vi "EAGLE Setup Screen V2.vi"() -> (1 "Table Control":string[][](table))   [LabVIEW 2015]
panel:
  in  "AvgPuls":dbl=0.3 min=0.3 max=2.0 format="%#.2g"
  in  "DfromLim":dbl min=-1000.0 max=1000.0
  in  "TbetweenP":u32=4 min=4 max=10
  in  "NumOfLas":u32=1 min=1 max=100
  in  "EyeColor":enum32{"Dark", "Blue/Green"}(radio) caption="Eye Color"
  in  "EyeSelect":enum32{"Right Eye", "Left Eye"}(radio) caption="Eye"
  in  "TreatArea":enum32{"Upper 180", "Lower 180", "Full 360"}(radio) caption="Treatment Area"
  in  "ID":string caption="Patient ID"
  in  "Save":bool
  in  "AvgPulseEn":dbl(slide)=1.0 caption="Average Pulse\nEnergy [mJ]" min=0.3 max=2.0 step=0.1 scale=0.3..2.0
  in  "DisFromLimbus":dbl(slide)=1.0 caption="Distance From \nLimbus [um]" min=-1000.0 max=1000.0 step=0.1 scale=-1000.0..1000.0
  in  "TBetweenPulses":u8(slide)=4 caption="Time Between \nPulses [mSec]" min=4 max=10 step=1 scale=4.0..10.0
  in  "LaserShots":u8(slide)=1 caption="Number of \nLaser Pulses" min=1 max=100 step=1 scale=1.0..100.0
  in  "FillSetupList":bool
  in  "Done":bool
  # "Treatment Settings"
  # "Laser Settings"
  # "Eye Info"
  # "Treatment Info"
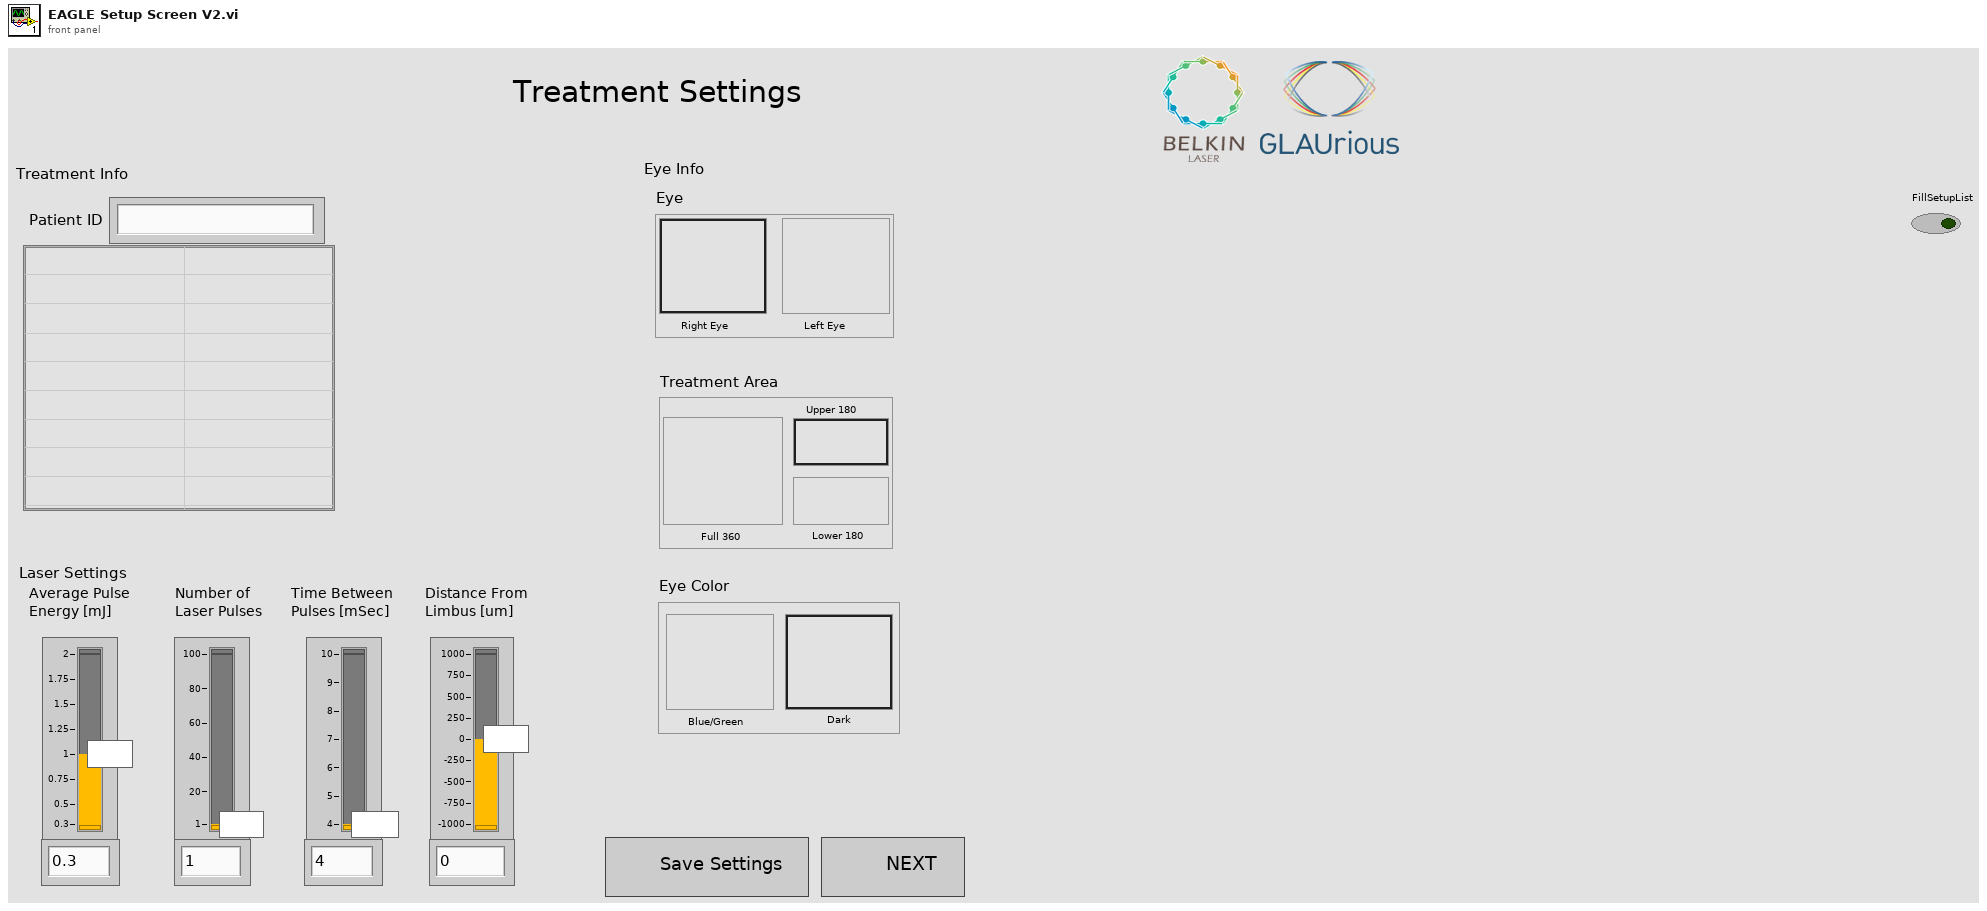
[diagram p1: front panel]
types:
  T1 = typedef "LVRectTypeDef.ctl" = cluster{"Left":i16, "Top":i16, "Right":i16, "Bottom":i16}
  T2 = typedef "LVPositionTypeDef.ctl" = cluster{"Left":i32, "Top":i32}
  T3 = cluster{"EyeSelect":enum32{"Right Eye", "Left Eye"}, "TBetweenPulses":u8, "LaserShots":u8, "TreatArea":enum32{"Upper 180", "Lower 180", "Full 360"}, "DisFromLimbus":dbl, "ID":string, "EyeColor":enum32{"Dark", "Blue/Green"}, "AvgPulseEn":dbl}
  T4 = cluster{"EyeSelect":enum32{"Right Eye", "Left Eye"}, "TBetweenPulses":u8, "LaserShots":u8, "TreatArea":enum32{"Upper 180", "Lower 180", "Full 360"}, "DisFromLimbus":dbl, "ID":string, "EyeColor":enum32{"Dark", "Blue/Green"}, "AvgPulse":dbl}
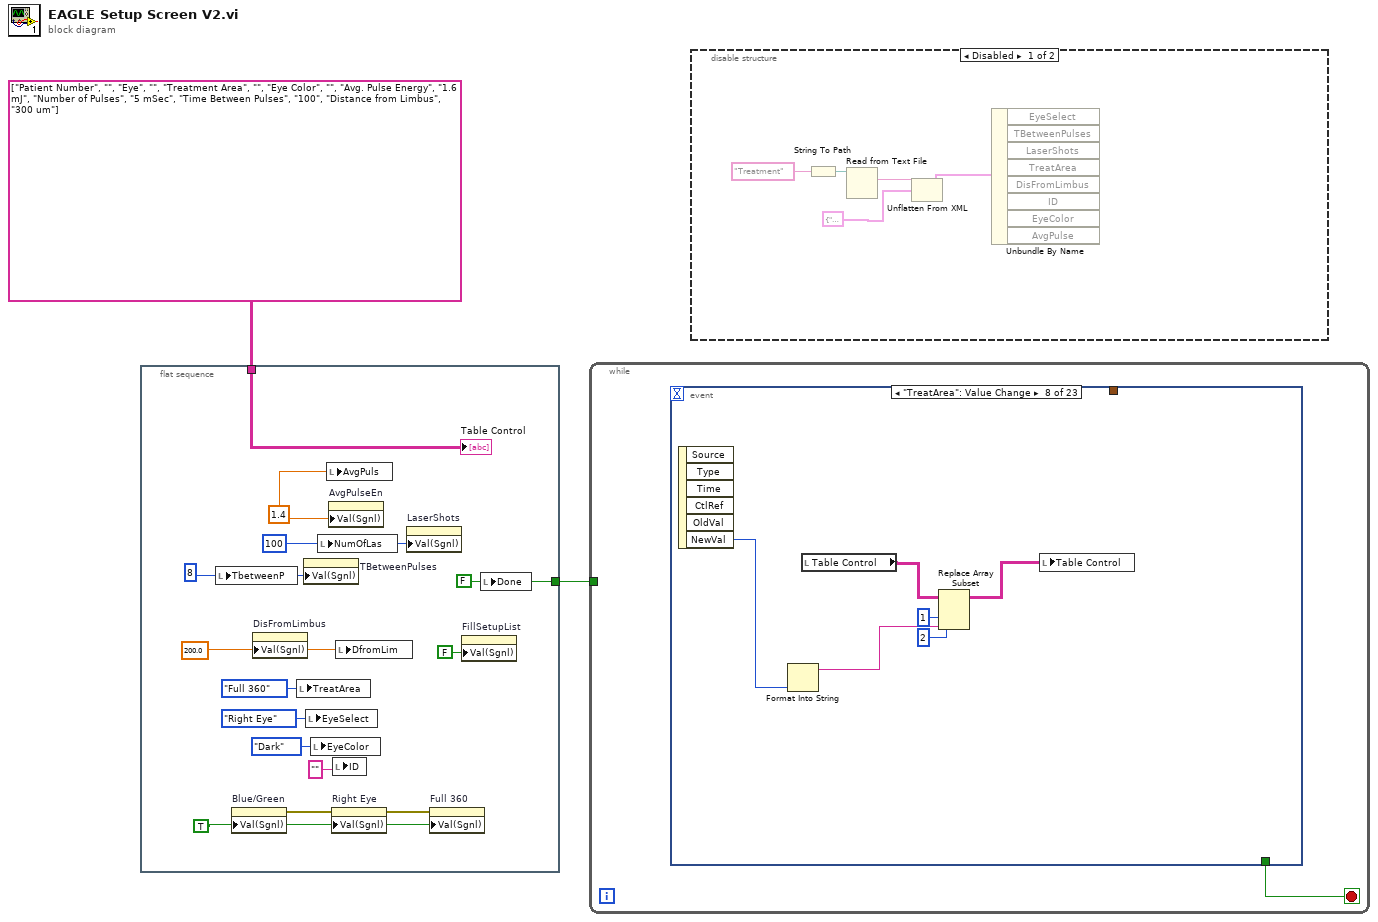
[diagram p0: block diagram]
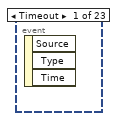
[diagram p3: hidden frame]
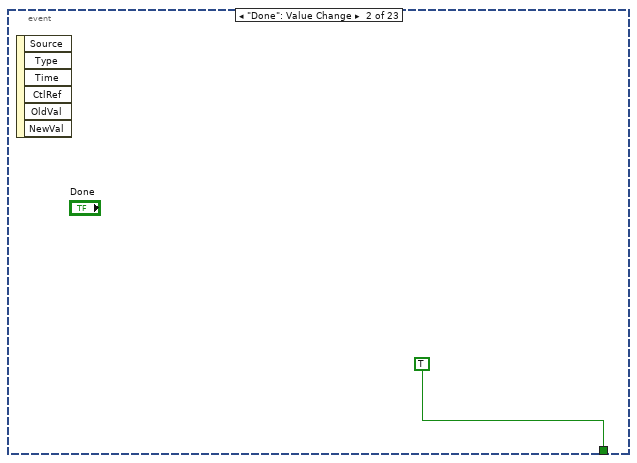
[diagram p4: hidden frame]
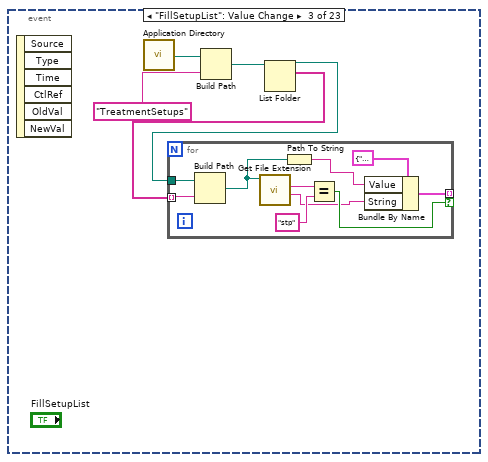
[diagram p5: hidden frame]
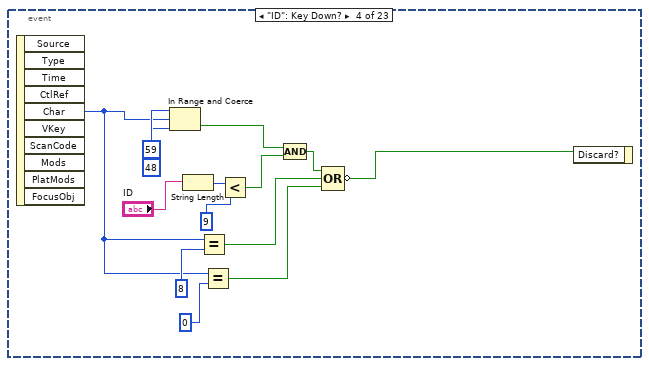
[diagram p6: hidden frame]
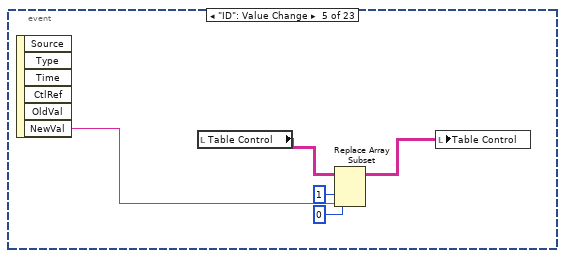
[diagram p7: hidden frame]
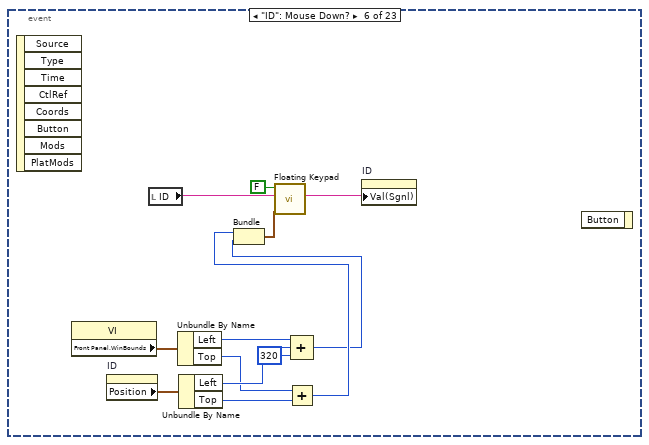
[diagram p8: hidden frame]
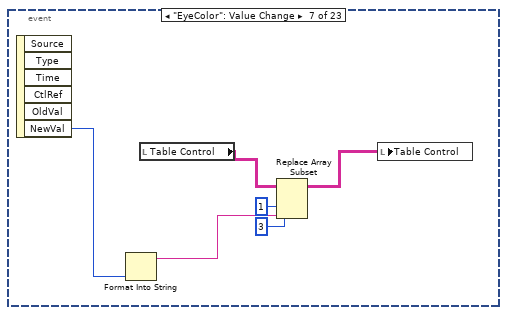
[diagram p9: hidden frame]
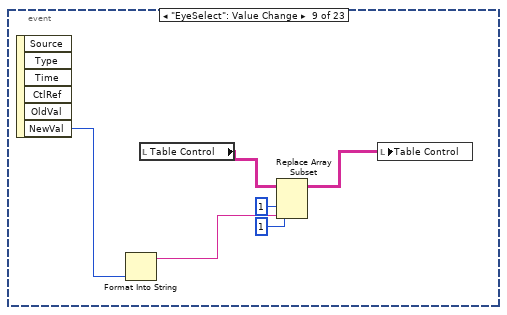
[diagram p10: hidden frame]
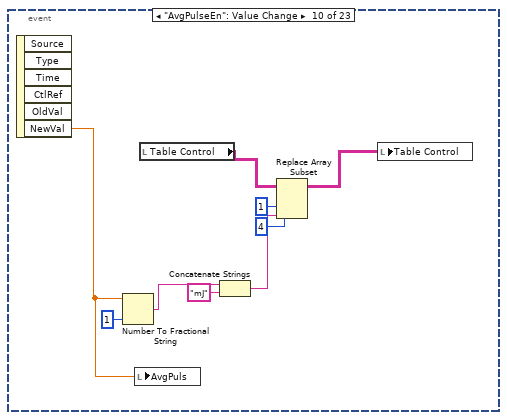
[diagram p11: hidden frame]
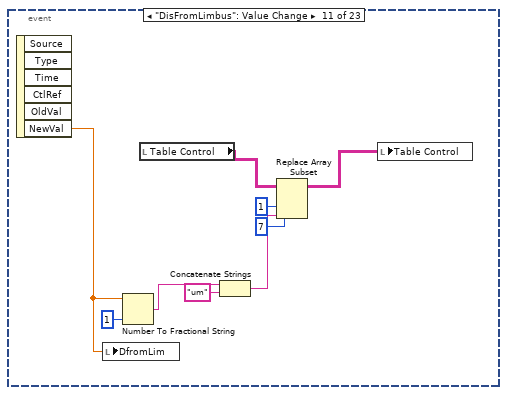
[diagram p12: hidden frame]
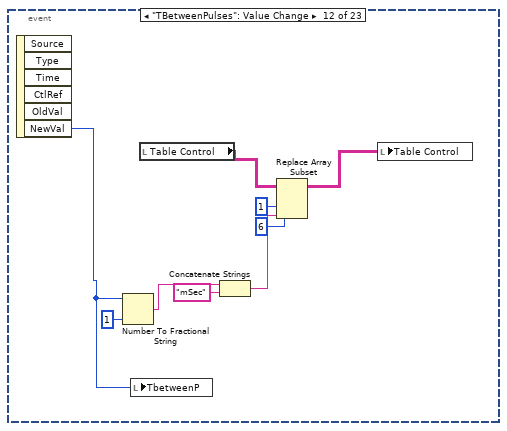
[diagram p13: hidden frame]
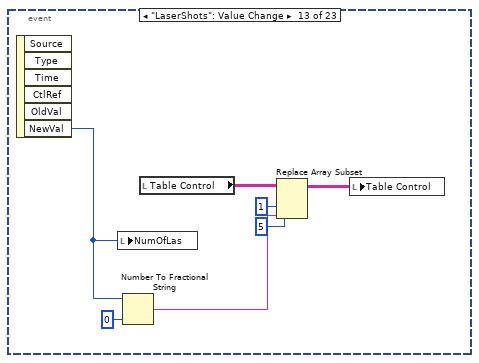
[diagram p14: hidden frame]
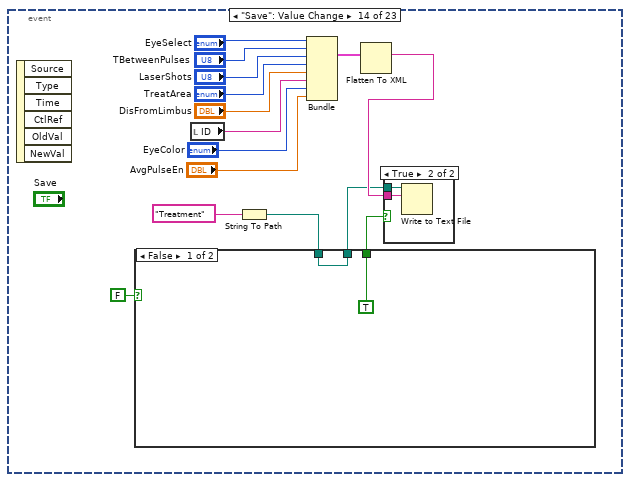
[diagram p15: hidden frame]
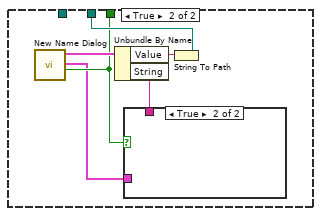
[diagram p17: hidden frame]
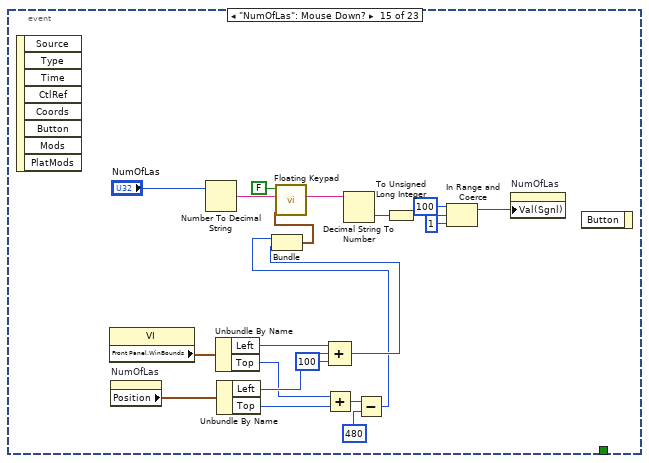
[diagram p19: hidden frame]
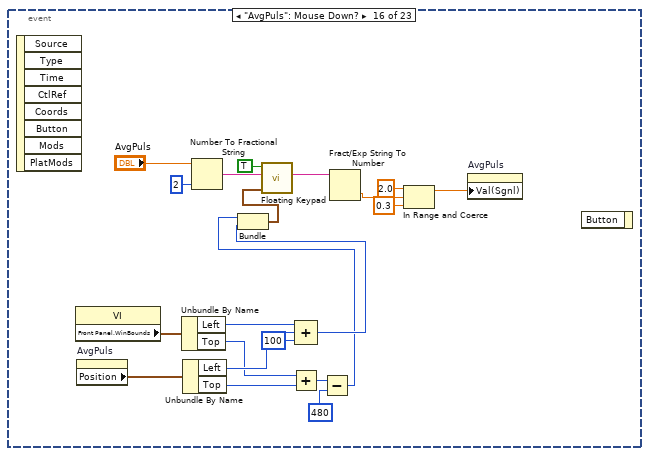
[diagram p20: hidden frame]
diagram:
  n1 = flat-sequence {
    tunnel: [w16] -> w2
    tunnel: string[][] [["Patient Number", ""], ["Eye", ""], ["Treatment Area", ""], ["Eye Color", ""], ["Avg. Pulse Energy", "1.6 mJ"], ["Number of Pulses", "5 mSec"], ["Time Between Pulses", "100"], ["Distance from Limbus", "300 um"]] ("Table Control") -> [w14]
    frame #0 {
      w3 = TRUE
      w6 = 200.0 ("DisFromLimbus")
      w7 = u8 8 ("TBetweenPulses")
      w8 = u8 100 ("LaserShots")
      w9 = 1.4 ("AvgPulse")
      w16 = FALSE ("Done")
      n2 = local write "TbetweenP"(w7) -> ()
      n3 = property on="Blue/Green" class="Bool (strict)"("Val(Sgnl)"=w3) -> (error out=w5:errorcluster)  [unwired: 2 in, 1 out]
      n4 = property on="DisFromLimbus" class="Slide (strict)"("Val(Sgnl)"=w6) -> ()  [unwired: 2 in, 2 out]
      n5 = local write "TreatArea"(enum32{"Upper 180", "Lower 180", "Full 360"}."Full 360" ("TreatArea")) -> ()
      n6 = property on="TBetweenPulses" class="Slide (strict)"("Val(Sgnl)"=w7) -> ()  [unwired: 2 in, 2 out]
      n7 = local write "EyeSelect"(enum32{"Right Eye", "Left Eye"}."Right Eye" ("EyeSelect")) -> ()
      n8 = local write "EyeColor"(enum32{"Dark", "Blue/Green"}."Dark" ("EyeColor")) -> ()
      n9 = local write "NumOfLas"(w8) -> ()
      n10 = local write "AvgPuls"(w9) -> ()
      n11 = property on="AvgPulseEn" class="Slide (strict)"("Val(Sgnl)"=w9) -> ()  [unwired: 2 in, 2 out]
      n12 = property on="Right Eye" class="Bool (strict)"(error in=w5, "Val(Sgnl)"=w3) -> (error out=w4:errorcluster)  [unwired: 1 in, 1 out]
      n13 = local write "ID"("" ("ID")) -> ()
      n14 = local write "DfromLim"(w6) -> ()
      n15 = property on="LaserShots" class="Slide (strict)"("Val(Sgnl)"=w8) -> ()  [unwired: 2 in, 2 out]
      n16 = property on="Full 360" class="Bool (strict)"(error in=w4, "Val(Sgnl)"=w3) -> ()  [unwired: 1 in, 2 out]
      n17 = property on="FillSetupList" class="Bool (strict)"("Val(Sgnl)"=FALSE ("Value (Signaling)")) -> ()  [unwired: 2 in, 2 out]
      n18 = local write "Done"(w16) -> ()
      "Table Control" <- w14
    }
  }
  n19 = while {
    tunnel: w2 -> [_]
    stop <- w17 stop-if-true
    n20 = event shown="[7] \"TreatArea\": Value Change" {
      selector: _ -> [_ _ _ _ _ _ _ _ _ _ _ _ _ _ _ _ _ _ _ _ _ _ _]
      dyn-events: _ -> [_ _ _ _ _ _ _ _ _ _ _ _ _ _ _ _ _ _ _ _ _ _ _]
      timeout: _ -> [_ _ _ _ _ _ _ _ _ _ _ _ _ _ _ _ _ _ _ _ _ _ _]
      tunnel: [_ TRUE _ _ _ _ _ _ _ _ _ _ _ _ _ _ _ _ _ _ _ _ _] -> w17
      tunnel: [_ _ _ _ _ _ _ _ _ _ _ _ _ _ _ _ _ _ _ _ w226 _ _] -> _
      event Timeout {
        n21 = event-data() -> ()  [unwired: 1 in, 3 out]
      }
      event "Done": Value Change {
        n22 = event-data() -> ()  [unwired: 1 in, 6 out]
      }
      event "FillSetupList": Value Change {
        n23 = event-data() -> ()  [unwired: 1 in, 6 out]
        n24 = call <vilib>:"Application Directory.vi"() -> ("Application Directory"=w23:path)
        n25 = Build Path(base path=w23, name or relative path="TreatmentSetups") -> (appended path=w21:path)
        n26 = List Folder(path=w21) -> (path out=w19:path, filenames=w20:string[])  [unwired: 3 in, 2 out]
        n27 = for {
          tunnel: w20 -> [w28] mode=indexing
          tunnel: w19 -> [w33]
          tunnel: [w27] -> _ mode=indexing if=w26
          n28 = Build Path(base path=w33, name or relative path=w28) -> (appended path=w31:path)
          n29 = call <vilib>:"Get File Extension.vi"("file"=w31) -> ("filename without extension"=w24:string, "lowercase file extension"=w25:string)  [unwired: 6 in, 3 out]
          n30 = Path To String(path=w31) -> (string=w29:string)
          n31 = Equal?(x=w25, y="stp") -> (x = y?=w26:bool)
          n32 = Bundle By Name(cluster=cluster{"String":string, "Value":string} {"String"="", "Value"=""}, "Value"=w29, "String"=w24) -> (w27:cluster{"String":string, "Value":string})
        }
      }
      event "ID": Key Down? {
        n33 = event-data() -> ("Char"=w39:i16)  [unwired: 1 in, 9 out]
        n34 = In Range and Coerce(upper limit=i16 59, x=w39, lower limit=i16 48) -> (In Range?=w42:bool)  [unwired: 1 out]
        n35 = String Length(string="ID") -> (length=w44:i32)
        n36 = Equal?(x=w39, y=i16 8) -> (x = y?=w36:bool)
        n37 = Equal?(x=w39, y=i16 0) -> (x = y?=w35:bool)
        n38 = Less?(x=w44, y=9) -> (x < y?=w41:bool)
        n39 = Compound Arithmetic op=AND(w42, w41) -> (w37:bool)
        n40 = Compound Arithmetic op=OR(w37, w36, w35) -> (invert w34:bool)
        n41 = event-data("Discard?"=w34) -> ()  [unwired: 1 in, 1 out]
      }
      event "ID": Value Change {
        n42 = event-data() -> ("NewVal"=w48:string)  [unwired: 1 in, 5 out]
        n43 = local read "Table Control"() -> (w52:string[][])
        n44 = Replace Array Subset(array=w52, new element=w48, index (row)=0 ("disabled index (row)"), index (col)=1 ("disabled index (col)")) -> (w51:string[][])
        n45 = local write "Table Control"(w51) -> ()
      }
      event "ID": Mouse Down? {
        n46 = event-data() -> ()  [unwired: 1 in, 8 out]
        n47 = property class="VI"() -> ("Front Panel.WinBounds"=w62:T1)  [unwired: 2 in, 2 out]
        n48 = property on="ID" class="Str"() -> ("Position"=w61:T2)  [unwired: 2 in, 2 out]
        n49 = local read "ID"() -> (w65:string)
        n50 = Unbundle By Name(w62) -> ("Left"=w60:i16, "Top"=w57:i16)
        n51 = Unbundle By Name(w61) -> ("Left"=w59:i32, "Top"=w58:i32)
        n52 = Add(x=w57, y=w58) -> (x+y=w56:i32)
        n53 = Compound Arithmetic op=ADD(w60, w59, 320 ("value")) -> (w55:i32)
        n54 = Bundle(w56, w55) -> (w54:cluster{i32, i32})  [unwired: 1 in]
        n55 = call "Floating Keypad.vi"("Position"=w54, "StringIn"=w65, "Allow dot"=FALSE) -> ("StringOut"=w63:string)  [unwired: 8 in]
        n56 = property on="ID" class="Str"("Val(Sgnl)"=w63) -> ()  [unwired: 2 in, 2 out]
        n57 = event-data() -> ()  [unwired: 2 in, 1 out]
      }
      event "EyeColor": Value Change {
        n58 = event-data() -> ("NewVal"=w68:enum32{"Dark", "Blue/Green"})  [unwired: 1 in, 5 out]
        n59 = Format Into String(w68) -> (resulting string=w67:string)  [unwired: 3 in, 1 out]
        n60 = local read "Table Control"() -> (w71:string[][])
        n61 = Replace Array Subset(array=w71, new element=w67, index (row)=3 ("disabled index (row)"), index (col)=1 ("disabled index (col)")) -> (w70:string[][])
        n62 = local write "Table Control"(w70) -> ()
      }
      event "TreatArea": Value Change {
        n63 = event-data() -> ("NewVal"=w74:enum32{"Upper 180", "Lower 180", "Full 360"})  [unwired: 1 in, 5 out]
        n64 = Format Into String(w74) -> (resulting string=w73:string)  [unwired: 3 in, 1 out]
        n65 = local read "Table Control"() -> (w77:string[][])
        n66 = Replace Array Subset(array=w77, new element=w73, index (row)=2 ("disabled index (row)"), index (col)=1 ("disabled index (col)")) -> (w76:string[][])
        n67 = local write "Table Control"(w76) -> ()
      }
      event "EyeSelect": Value Change {
        n68 = event-data() -> ("NewVal"=w80:enum32{"Right Eye", "Left Eye"})  [unwired: 1 in, 5 out]
        n69 = Format Into String(w80) -> (resulting string=w79:string)  [unwired: 3 in, 1 out]
        n70 = local read "Table Control"() -> (w83:string[][])
        n71 = Replace Array Subset(array=w83, new element=w79, index (row)=1 ("disabled index (row)"), index (col)=1 ("disabled index (col)")) -> (w82:string[][])
        n72 = local write "Table Control"(w82) -> ()
      }
      event "AvgPulseEn": Value Change {
        n73 = event-data() -> ("NewVal"=w84:dbl)  [unwired: 1 in, 5 out]
        n74 = Number To Fractional String(number=w84, precision (6)=i16 1) -> (F-format string=w85:string)  [unwired: 2 in]
        n75 = local write "AvgPuls"(w84) -> ()
        n76 = local read "Table Control"() -> (w92:string[][])
        n77 = Concatenate Strings(w85, "mJ" ("string")) -> (w87:string)
        n78 = Replace Array Subset(array=w92, new element=w87, index (row)=4 ("disabled index (row)"), index (col)=1 ("disabled index (col)")) -> (w91:string[][])
        n79 = local write "Table Control"(w91) -> ()
      }
      event "DisFromLimbus": Value Change {
        n80 = event-data() -> ("NewVal"=w93:dbl)  [unwired: 1 in, 5 out]
        n81 = local write "DfromLim"(w93) -> ()
        n82 = Number To Fractional String(number=w93, precision (6)=i16 1) -> (F-format string=w94:string)  [unwired: 2 in]
        n83 = local read "Table Control"() -> (w101:string[][])
        n84 = Concatenate Strings(w94, "um" ("string")) -> (w96:string)
        n85 = Replace Array Subset(array=w101, new element=w96, index (row)=7 ("disabled index (row)"), index (col)=1 ("disabled index (col)")) -> (w100:string[][])
        n86 = local write "Table Control"(w100) -> ()
      }
      event "TBetweenPulses": Value Change {
        n87 = event-data() -> ("NewVal"=w102:u8)  [unwired: 1 in, 5 out]
        n88 = Number To Fractional String(number=w102, precision (6)=i16 1) -> (F-format string=w103:string)  [unwired: 2 in]
        n89 = local write "TbetweenP"(w102) -> ()
        n90 = local read "Table Control"() -> (w110:string[][])
        n91 = Concatenate Strings(w103, "mSec" ("string")) -> (w105:string)
        n92 = Replace Array Subset(array=w110, new element=w105, index (row)=6 ("disabled index (row)"), index (col)=1 ("disabled index (col)")) -> (w109:string[][])
        n93 = local write "Table Control"(w109) -> ()
      }
      event "LaserShots": Value Change {
        n94 = event-data() -> ("NewVal"=w111:u8)  [unwired: 1 in, 5 out]
        n95 = local write "NumOfLas"(w111) -> ()
        n96 = Number To Fractional String(number=w111, precision (6)=i16 0) -> (F-format string=w112:string)  [unwired: 2 in]
        n97 = local read "Table Control"() -> (w117:string[][])
        n98 = Replace Array Subset(array=w117, new element=w112, index (row)=5 ("disabled index (row)"), index (col)=1 ("disabled index (col)")) -> (w116:string[][])
        n99 = local write "Table Control"(w116) -> ()
      }
      event "Save": Value Change {
        n100 = event-data() -> ()  [unwired: 1 in, 6 out]
        n101 = local read "ID"() -> (w122:string)
        n102 = String To Path(string="Treatment") -> (path=w125:path)
        n103 = case shown="False" FALSE {
          tunnel: w125 -> [w136 _]
          tunnel: [w136 w140] -> w124
          tunnel: [TRUE w139] -> w123
          frame False {
          }
          frame True {
            n104 = call "New Name Dialog.vi"() -> ("OK"=w139:bool, "NamesOut"=w138:cluster{"String":string, "Value":string}[], "NewName"=w142:cluster{"String":string, "Value":string})  [unwired: 9 in]
            n105 = Unbundle By Name(w142) -> ("Value"=w141:string, "String"=w137:string)
            n106 = case shown="True" w139 {
              tunnel: w138 -> [_ _]
              tunnel: w137 -> [_ _]
              frame False {
              }
              frame True {
              }
            }
            n107 = String To Path(string=w141) -> (path=w140:path)
          }
        }
        n108 = Bundle("EyeSelect"="EyeSelect", "TBetweenPulses"="TBetweenPulses", "LaserShots"="LaserShots", "TreatArea"="TreatArea", "DisFromLimbus"="DisFromLimbus", "ID"=w122, "EyeColor"="EyeColor", "AvgPulseEn"="AvgPulseEn") -> (w132:T3)  [unwired: 1 in]
        n109 = Flatten To XML(anything=w132) -> (xml string=w126:string)
        n110 = case shown="True" w123 {
          tunnel: w126 -> [_ w134]
          tunnel: w124 -> [_ w133]
          frame False {
          }
          frame True {
            n111 = Write to Text File(file (use dialog)=w133, text=w134) -> ()  [unwired: 2 in, 3 out]
          }
        }
      }
      event "NumOfLas": Mouse Down? {
        n112 = event-data() -> ()  [unwired: 1 in, 8 out]
        n113 = property class="VI"() -> ("Front Panel.WinBounds"=w158:T1)  [unwired: 2 in, 2 out]
        n114 = property on="NumOfLas" class="DigNum (strict)"() -> ("Position"=w152:T2)  [unwired: 2 in, 2 out]
        n115 = Number To Decimal String(number="NumOfLas") -> (decimal integer string=w163:string)  [unwired: 1 in]
        n116 = Unbundle By Name(w158) -> ("Left"=w157:i16, "Top"=w154:i16)
        n117 = Unbundle By Name(w152) -> ("Left"=w156:i32, "Top"=w155:i32)
        n118 = Add(x=w154, y=w155) -> (x+y=w150:i32)
        n119 = Compound Arithmetic op=ADD(w157, w156, 100 ("value")) -> (w151:i32)
        n120 = Subtract(x=w150, y=480) -> (x-y=w148:i32)
        n121 = Bundle(w148, w151) -> (w147:cluster{i32, i32})  [unwired: 1 in]
        n122 = call "Floating Keypad.vi"("Position"=w147, "StringIn"=w163, "Allow dot"=FALSE) -> ("StringOut"=w162:string)  [unwired: 8 in]
        n123 = Decimal String To Number(string=w162) -> (number=w161:i32)  [unwired: 2 in, 1 out]
        n124 = To Unsigned Long Integer(number=w161) -> (unsigned 32bit integer=w146:u32)
        n125 = In Range and Coerce(upper limit=u32 100, x=w146, lower limit=u32 1) -> (coerced(x)=w145:u32)  [unwired: 1 out]
        n126 = property on="NumOfLas" class="DigNum (strict)"("Val(Sgnl)"=w145) -> ()  [unwired: 2 in, 2 out]
        n127 = event-data() -> ()  [unwired: 2 in, 1 out]
      }
      event "AvgPuls": Mouse Down? {
        n128 = event-data() -> ()  [unwired: 1 in, 8 out]
        n129 = property class="VI"() -> ("Front Panel.WinBounds"=w180:T1)  [unwired: 2 in, 2 out]
        n130 = property on="AvgPuls" class="DigNum (strict)"() -> ("Position"=w169:T2)  [unwired: 2 in, 2 out]
        n131 = Unbundle By Name(w180) -> ("Left"=w179:i16, "Top"=w176:i16)
        n132 = Unbundle By Name(w169) -> ("Left"=w178:i32, "Top"=w177:i32)
        n133 = Number To Fractional String(number="AvgPuls", precision (6)=i16 2) -> (F-format string=w184:string)  [unwired: 2 in]
        n134 = Add(x=w176, y=w177) -> (x+y=w173:i32)
        n135 = Compound Arithmetic op=ADD(w179, w178, 100 ("value")) -> (w174:i32)
        n136 = Subtract(x=w173, y=480) -> (x-y=w171:i32)
        n137 = Bundle(w171, w174) -> (w170:cluster{i32, i32})  [unwired: 1 in]
        n138 = call "Floating Keypad.vi"("Position"=w170, "StringIn"=w184, "Allow dot"=TRUE) -> ("StringOut"=w183:string)  [unwired: 8 in]
        n139 = Fract/Exp String To Number(string=w183) -> (number=w166:dbl)  [unwired: 3 in, 1 out]
        n140 = In Range and Coerce(upper limit=2.0, x=w166, lower limit=0.3) -> (coerced(x)=w167:dbl)  [unwired: 1 out]
        n141 = property on="AvgPuls" class="DigNum (strict)"("Val(Sgnl)"=w167) -> ()  [unwired: 2 in, 2 out]
        n142 = event-data() -> ()  [unwired: 2 in, 1 out]
      }
      event "AvgPuls": Value Change {
        n143 = event-data() -> ("NewVal"=w185:dbl)  [unwired: 1 in, 5 out]
        n144 = property on="AvgPulseEn" class="Slide (strict)"("Val(Sgnl)"=w185) -> ()  [unwired: 2 in, 2 out]
      }
      event "NumOfLas": Value Change {
        n145 = event-data() -> ("NewVal"=w186:u32)  [unwired: 1 in, 5 out]
        n146 = property on="LaserShots" class="Slide (strict)"("Val(Sgnl)"=w186) -> ()  [unwired: 2 in, 2 out]
      }
      event "TbetweenP": Mouse Down? {
        n147 = event-data() -> ()  [unwired: 1 in, 8 out]
        n148 = property class="VI"() -> ("Front Panel.WinBounds"=w202:T1)  [unwired: 2 in, 2 out]
        n149 = property on="TbetweenP" class="DigNum (strict)"() -> ("Position"=w191:T2)  [unwired: 2 in, 2 out]
        n150 = Unbundle By Name(w202) -> ("Left"=w201:i16, "Top"=w198:i16)
        n151 = Unbundle By Name(w191) -> ("Left"=w200:i32, "Top"=w199:i32)
        n152 = Number To Decimal String(number="TbetweenP") -> (decimal integer string=w207:string)  [unwired: 1 in]
        n153 = Add(x=w198, y=w199) -> (x+y=w195:i32)
        n154 = Compound Arithmetic op=ADD(w201, w200, 100 ("value")) -> (w196:i32)
        n155 = Subtract(x=w195, y=480) -> (x-y=w193:i32)
        n156 = Bundle(w193, w196) -> (w192:cluster{i32, i32})  [unwired: 1 in]
        n157 = call "Floating Keypad.vi"("Position"=w192, "StringIn"=w207, "Allow dot"=FALSE) -> ("StringOut"=w206:string)  [unwired: 8 in]
        n158 = Decimal String To Number(string=w206) -> (number=w205:i32)  [unwired: 2 in, 1 out]
        n159 = To Unsigned Long Integer(number=w205) -> (unsigned 32bit integer=w190:u32)
        n160 = In Range and Coerce(upper limit=u32 10, x=w190, lower limit=u32 4) -> (coerced(x)=w189:u32)  [unwired: 1 out]
        n161 = property on="TbetweenP" class="DigNum (strict)"("Val(Sgnl)"=w189) -> ()  [unwired: 2 in, 2 out]
        n162 = event-data() -> ()  [unwired: 2 in, 1 out]
      }
      event "TbetweenP": Value Change {
        n163 = event-data() -> ("NewVal"=w208:u32)  [unwired: 1 in, 5 out]
        n164 = property on="TBetweenPulses" class="Slide (strict)"("Val(Sgnl)"=w208) -> ()  [unwired: 2 in, 2 out]
      }
      event "DfromLim": Mouse Down? {
        n165 = event-data() -> ()  [unwired: 1 in, 8 out]
        n166 = property class="VI"() -> ("Front Panel.WinBounds"=w225:T1)  [unwired: 2 in, 2 out]
        n167 = property on="DfromLim" class="DigNum (strict)"() -> ("Position"=w214:T2)  [unwired: 2 in, 2 out]
        n168 = property on="DfromLim" class="DigNum (strict)"() -> ("Position"=w226:T2)  [unwired: 2 in, 2 out]
        n169 = Number To Fractional String(number="DfromLim", precision (6)=i16 1) -> (F-format string=w229:string)  [unwired: 2 in]
        n170 = Unbundle By Name(w225) -> ("Left"=w224:i16, "Top"=w221:i16)
        n171 = Unbundle By Name(w214) -> ("Left"=w223:i32, "Top"=w222:i32)
        n172 = Add(x=w221, y=w222) -> (x+y=w218:i32)
        n173 = Compound Arithmetic op=ADD(w224, w223, 100 ("value")) -> (w219:i32)
        n174 = Subtract(x=w218, y=480) -> (x-y=w216:i32)
        n175 = Bundle(w216, w219) -> (w215:cluster{i32, i32})  [unwired: 1 in]
        n176 = call "Floating Keypad.vi"("Position"=w215, "StringIn"=w229, "Allow dot"=TRUE) -> ("StringOut"=w228:string)  [unwired: 8 in]
        n177 = Fract/Exp String To Number(string=w228) -> (number=w212:dbl)  [unwired: 3 in, 1 out]
        n178 = In Range and Coerce(upper limit=1000.0, x=w212, lower limit=-1000.0) -> (coerced(x)=w211:dbl)  [unwired: 1 out]
        n179 = property on="DfromLim" class="DigNum (strict)"("Val(Sgnl)"=w211) -> ()  [unwired: 2 in, 2 out]
        n180 = event-data() -> ()  [unwired: 2 in, 1 out]
      }
      event "DfromLim": Value Change {
        n181 = event-data() -> ("NewVal"=w231:dbl)  [unwired: 1 in, 5 out]
        n182 = property on="DisFromLimbus" class="Slide (strict)"("Val(Sgnl)"=w231) -> ()  [unwired: 2 in, 2 out]
      }
      event Panel Close? {
        n183 = event-data() -> ()  [unwired: 1 in, 4 out]
        n184 = property on="Done" class="Bool (strict)"("Val(Sgnl)"=FALSE ("Value (Signaling)")) -> ()  [unwired: 2 in, 2 out]
        n185 = event-data("Discard?"=TRUE) -> ()  [unwired: 1 in, 1 out]
      }
    }
  }
  n186 = disable-structure shown="Disabled" {
    frame Disabled {
      n187 = String To Path(string="Treatment") -> (path=w234:path)
      n188 = Read from Text File(file (use dialog)=w234) -> (text=w235:string)  [unwired: 3 in, 3 out]
      n189 = Unflatten From XML(xml string=w235, type=T4 {"EyeSelect"=enum."Right Eye", "TBetweenPulses"=0, "LaserShots"=0, "TreatArea"=enum."Upper 180", "DisFromLimbus"=0.0, "ID"="", "EyeColor"=enum."Dark", "AvgPulse"=0.0} ("output cluster")) -> (value=w236:T4)  [unwired: 1 in, 1 out]
      n190 = Unbundle By Name(w236) -> ("EyeSelect"=w237:enum32{"Right Eye", "Left Eye"}, "TBetweenPulses"=w238:u8, "LaserShots"=w239:u8, "TreatArea"=w240:enum32{"Upper 180", "Lower 180", "Full 360"}, "DisFromLimbus"=w241:dbl, "EyeColor"=w242:enum32{"Dark", "Blue/Green"}, "AvgPulse"=w244:dbl)  [unwired: 1 out]
    }
    frame Enabled {
    }
  }
